vi "Create.vi"(8 "error in (no error)":errorcluster) -> (0 "error out":errorcluster, 3 "Store out":refnum<class "Store.lvclass">)   [LabVIEW 2018, in "Application.lvlib" / "Store.lvclass"]
uses:
  Store.lvclass
  Store.lvclass/Store.ctl
  Dictionary Class/Dictionary.lvclass
panel:
  in  "Store in":refnum<class "Store.lvclass">
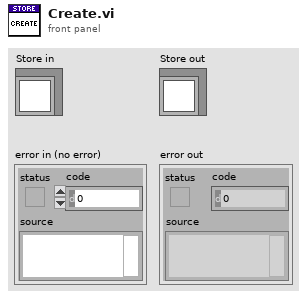
[diagram p1: front panel]
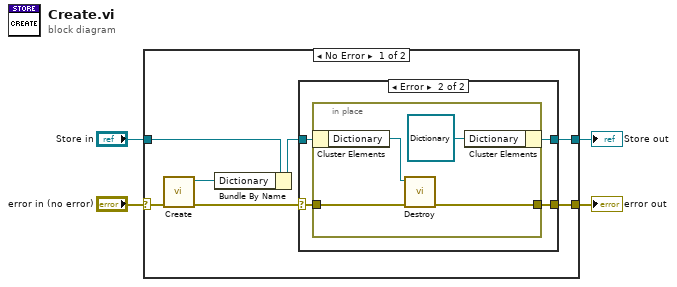
[diagram p0: block diagram]
diagram:
  n1 = case shown="No Error" "error in (no error)" {
    selector: "error in (no error)" -> [w10 w23]
    tunnel: [w5 w23] -> w3
    tunnel: [w6 w22] -> w1
    tunnel: "Store in" -> [w11 w22]
    frame No Error {
      n2 = call "Create.vi"("error in (no error)"=w10) -> ("error out"=w8:errorcluster, "Dictionary out"=w9:refnum<class "Dictionary.lvclass">)  [unwired: 9 in]
      n3 = Bundle By Name(cluster=w11, "Dictionary"=w9) -> (w7:refnum<class "Store.lvclass">)
      n4 = case shown="Error" w8 {
        selector: w8 -> [w12 w17]
        tunnel: w7 -> [w13 w16]
        tunnel: [w13 w15] -> w6
        tunnel: [w12 w14] -> w5
        frame No Error {
        }
        frame Error {
          n5 = in-place {
            in-place-border: w17 -> [w21]
            in-place-border: [w18] -> w14
            n6 = in-place-cluster #1(w16) -> ("Dictionary"=w20:refnum<class "Dictionary.lvclass">)
            n7 = call "Destroy.vi"("error in (no error)"=w21, "Dictionary in"=w20) -> ("error out"=w18:errorcluster)  [unwired: 7 in, 2 out]
            n8 = in-place-cluster #1("Dictionary"=refnum<class "Dictionary.lvclass"> refnum) -> (w15:refnum<class "Store.lvclass">)
          }
        }
      }
    }
    frame Error {
    }
  }
  "error out" <- w3
  "Store out" <- w1
